vi "Write.vi"(8 "error in (no error)":errorcluster, 10 "write buffer":string, 11 "MODBUS in":refnum<class "Modbus.lvclass">) -> (0 "error out":errorcluster, 3 "MODBUS Out":refnum<class "Modbus.lvclass">)   [LabVIEW 2020, in "Library Instrument & Equipement.lvlib" / "Library Relay_Board.lvlib" / "Modbus.lvclass"]
doc: "Writes bytes to specified interface."
uses:
  Modbus.lvclass
  Modbus.lvclass/Modbus.ctl
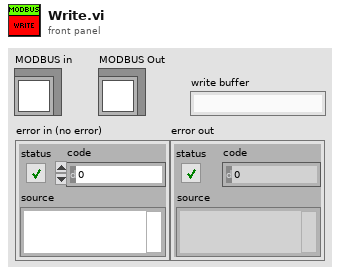
[diagram p1: front panel]
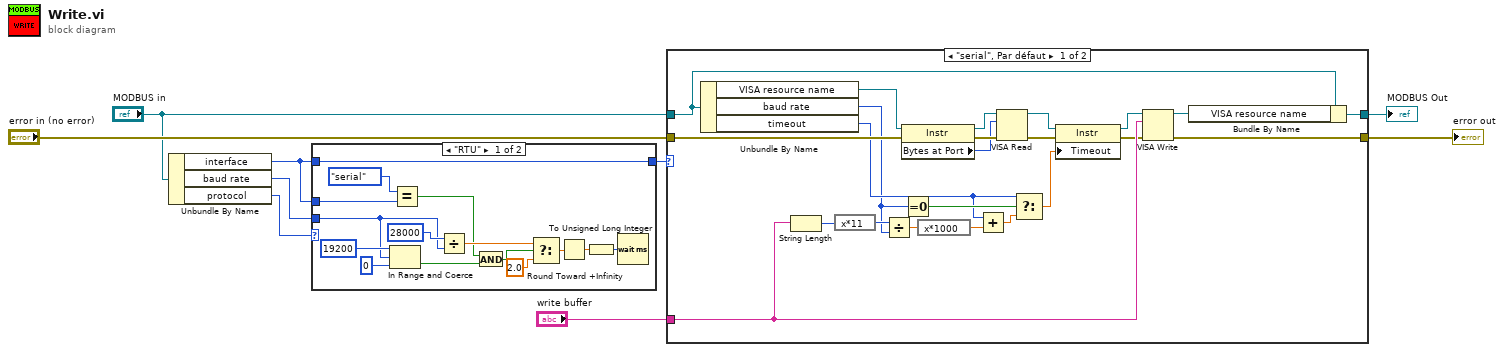
[diagram p0: block diagram]
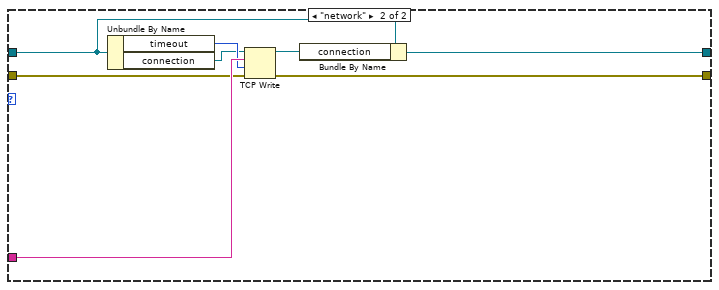
[diagram p3: hidden frame]
diagram:
  n1 = Unbundle By Name("MODBUS in") -> ("interface"=w4:enum16{"serial", "network"}, "baud rate"=w5:u32, "protocol"=w6:enum16{"RTU", "ASCII", "TCP"})
  n2 = case shown="\"RTU\"" w6 {
    tunnel: w5 -> [w14 _]
    tunnel: w4 -> [w13 _]
    tunnel: w4 -> [w11 w25]
    tunnel: [w11 w25] -> w3
    frame "RTU" {
      n3 = In Range and Coerce(upper limit=u32 19200, x=w14, lower limit=u32 0) -> (In Range?=w16:bool)  [unwired: 1 out]
      n4 = Equal?(x=enum16{"serial", "TCP"}."serial", y=w13) -> (x = y?=w17:bool)
      n5 = Divide(x=u32 28000, y=w14) -> (x/y=w20:dbl)
      n6 = And(x=w17, y=w16) -> (x .and. y?=w15:bool)
      n7 = Select(t=w20, s=w15, f=2.0) -> (s? t:f=w19:dbl)
      n8 = Round Toward +Infinity(x=w19) -> (ceil(x): smallest int >= x=w10:dbl)
      n9 = To Unsigned Long Integer(number=w10) -> (unsigned 32bit integer=w12:u32)
      n10 = Wait (ms)(milliseconds to wait=w12) -> ()  [unwired: 1 out]
    }
    frame "ASCII", Default {
    }
  }
  n11 = case shown="\"serial\", Par défaut" w3 {
    tunnel: "MODBUS in" -> [w48 w52]
    tunnel: "error in (no error)" -> [w40 w50]
    tunnel: [w46 w56] -> w9
    tunnel: [w45 w55] -> w8
    tunnel: "write buffer" -> [w34 w53]
    frame "serial", Default {
      n12 = Unbundle By Name(w48) -> ("VISA resource name"=w44:refnum<visa-resource-name>, "baud rate"=w31:u32, "timeout"=w32:u32)
      n13 = String Length(string=w34) -> (length=w33:i32)
      n14 = expression code="x*11"(w33) -> (w36:i32)
      n15 = Divide(x=w36, y=w31) -> (x/y=w37:dbl)
      n16 = property class="Instr"(reference=w44, error in=w40) -> (reference out=w43:refnum<visa-resource-name>, error out=w42:errorcluster, "Bytes at Port"=w41:u32)
      n17 = Equal To 0?(x=w31) -> (x = 0?=w35:bool)
      n18 = expression code="x*1000"(w37) -> (w39:dbl)
      n19 = Add(x=w32, y=w39) -> (x+y=w38:dbl)
      n20 = VISA Read(VISA resource name=w43, byte count=w41, error in (no error)=w42) -> (VISA resource name out=w29:refnum<visa-resource-name>, error out=w30:errorcluster)  [unwired: 2 out]
      n21 = Select(t=w32, s=w35, f=w38) -> (s? t:f=w26:dbl)
      n22 = property class="Instr"(reference=w29, error in=w30, "Timeout"=w26) -> (reference out=w28:refnum<visa-resource-name>, error out=w27:errorcluster)
      n23 = VISA Write(VISA resource name=w28, write buffer=w34, error in (no error)=w27) -> (VISA resource name out=w47:refnum<visa-resource-name>, error out=w45:errorcluster)  [unwired: 1 out]
      n24 = Bundle By Name(cluster=w48, "VISA resource name"=w47) -> (w46:refnum<class "Modbus.lvclass">)
    }
    frame "network" {
      n25 = Unbundle By Name(w52) -> ("timeout"=w51:u32, "connection"=w49:refnum<k5>)
      n26 = TCP Write(connection ID=w49, data in=w53, error in (no error)=w50, 9:w51) -> (connection ID out=w54:refnum<k5>, error out=w55:errorcluster)  [unwired: 1 out]
      n27 = Bundle By Name(cluster=w52, "connection"=w54) -> (w56:refnum<class "Modbus.lvclass">)
    }
  }
  "MODBUS Out" <- w9
  "error out" <- w8
